vi "ODSS_Msg.vi"(8 "error in":errorcluster, 11 "Msg":T1) -> (0 "error out":errorcluster)   [LabVIEW 2010]
doc: "This VI implements the routine for sending messages to the OpenDSS actor. This routine gets the queue of the OpenDSS actor and sends an \"exit\" Msg to the actor.\n\nCreated by Davis Montenegro\n06-30-2017"
uses:
  Ctrls/ODSS_Msgs.ctl
  Vars/Comm_Vars.vi
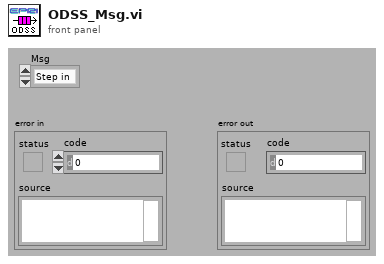
[diagram p1: front panel]
types:
  T1 = typedef "ODSS_Msgs.ctl" = enum16{"Step in", "Exit", "Sim Time", "Set Working Dir"}
  T2 = cluster{"actor_name":string, "actor_type":string, "queue":variant}[]
  T3 = cluster{"actor_name":string, "actor_type":string, "queue":variant}
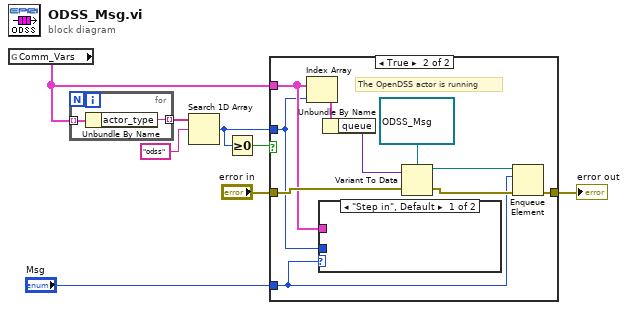
[diagram p0: block diagram]
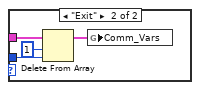
[diagram p3: hidden frame]
diagram:
  n1 = global read "Comm_Vars.vi" "Comm_Vars"() -> (w4:T2)
  n2 = for {
    tunnel: w4 -> [w10] mode=indexing
    tunnel: [w9] -> w5 mode=indexing
    n3 = Unbundle By Name(w10) -> ("actor_type"=w9:string)
  }
  n4 = Search 1D Array(1D array=w5, element="odss") -> (index of element=w3:i32)  [unwired: 1 in]
  n5 = Greater Or Equal To 0?(x=w3) -> (x >= 0?=w2:bool)
  n6 = case shown="True" w2 {
    tunnel: [w11 w20] -> w8
    tunnel: "error in" -> [w11 w18]
    tunnel: "Msg" -> [_ w15]
    tunnel: w4 -> [_ w14]
    tunnel: w3 -> [_ w13]
    frame False {
      # "The OpenDSS actor is not running, action cancelled"
    }
    frame True {
      w12 = refnum<queue> refnum items=["Step in", "Exit", "Sim Time", "Set Working Dir"] ("queue")
      # "The OpenDSS actor is running"
      n7 = Index Array(array=w14, index=w13) -> (element=w16:T3)
      n8 = case shown="\"Step in\", Default" w15 {
        tunnel: w14 -> [_ w25]
        tunnel: w13 -> [_ w24]
        frame "Step in", Default {
        }
        frame "Exit" {
          n9 = Delete From Array(array=w25, length=1, index=w24) -> (array with subset deleted=w22:T2)  [unwired: 1 out]
          n10 = global write "Comm_Vars.vi" "Comm_Vars"(w22) -> ()
        }
      }
      n11 = Unbundle By Name(w16) -> ("queue"=w17:variant)
      n12 = Variant To Data(error in=w18, Variant=w17, type=w12) -> (error out=w19:errorcluster, data=w21:refnum<queue>)
      n13 = Enqueue Element(queue=w21, element=w15, error in (no error)=w19) -> (error out=w20:errorcluster)  [unwired: 1 in, 2 out]
    }
  }
  "error out" <- w8
